vi "update.description.request.vi"(8 "error in":errorcluster, 10 "description":string, 11 "event":refnum<class "event.lvclass">) -> (0 "error out":errorcluster, 3 "request":string)   [LabVIEW 2020, in "event.lvclass"]
uses:
  event.lvclass
  event.lvclass/event.ctl
  ea825c25-c588-4097-8fc0-46daf0b2f069.vi
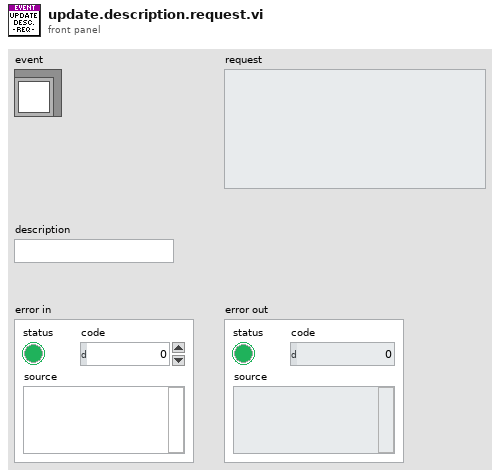
[diagram p1: front panel]
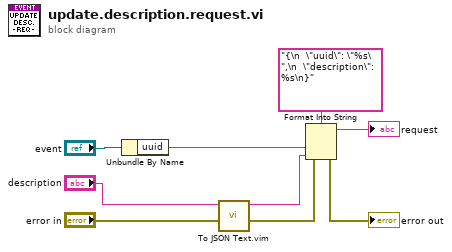
[diagram p0: block diagram]
diagram:
  n1 = Unbundle By Name("event") -> ("uuid"=w7:string)
  n2 = call "To JSON Text.vim"("error in (no error)"="error in", "Anything"="description") -> ("error out"=w3:errorcluster, "<JSON>"=w1:string)  [unwired: 8 in]
  n3 = Format Into String(format string="{\n  \"uuid\": \"%s\",\n  \"description\": %s\n}", error in=w3, w7, w1) -> (resulting string=→"request":string, error out=→"error out":errorcluster)  [unwired: 1 in]
